vi "Configure File.vi"(8 "Error In":errorcluster, 11 "Configuration":T1={"Root Folder"=path "", "Enable Calendar Tree"=TRUE, "Maximum File Size"=15728640, "Maximum File Count"=0, "File Extension"="csv"}) -> (0 "Error Out":errorcluster)   [LabVIEW 2017, in "Toolkit.lvlib"]
doc: "All of the configurations for the default log file can be configured with this one VI instead of using VIs for each individual configuration. The individual configuration VIs are just wrappers around this VI."
uses:
  Toolkit.lvlib
  Controls/Configuration.ctl
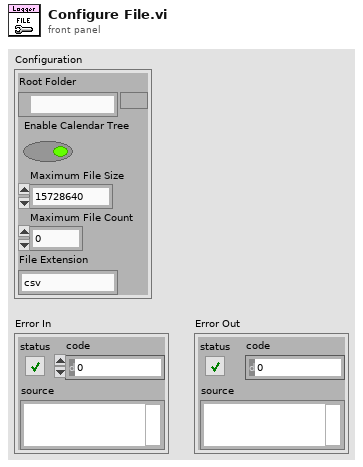
[diagram p1: front panel]
types:
  T1 = typedef "Toolkit.lvlib/Configuration.ctl" = cluster{"Root Folder":path, "Enable Calendar Tree":bool, "Maximum File Size":i64, "Maximum File Count":i32, "File Extension":string}
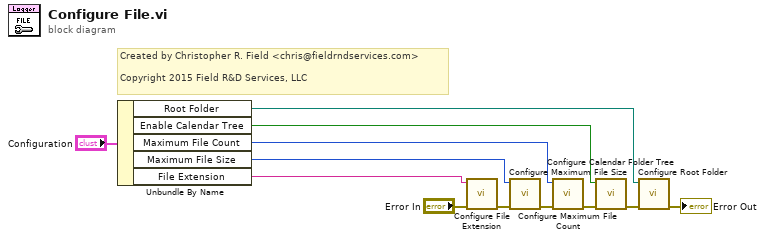
[diagram p0: block diagram]
diagram:
  # "Created by Christopher R. Field <chris@fieldrndservices.com>\n\nCopyright 2015 Field R&D Services, LLC"
  n1 = Unbundle By Name("Configuration") -> ("Root Folder"=w6:path, "Enable Calendar Tree"=w7:bool, "Maximum File Count"=w1:i32, "Maximum File Size"=w2:i64, "File Extension"=w8:string)
  n2 = call "Configure File Extension.vi"("Error In"="Error In", "File Extension"=w8) -> ("Error Out"=w3:errorcluster)  [unwired: 9 in]
  n3 = call "Configure Maximum File Size.vi"("Error In"=w3, "File Size"=w2) -> ("Error Out"=w4:errorcluster)  [unwired: 9 in]
  n4 = call "Configure Maximum File Count.vi"("Error In"=w4, "Maximum"=w1) -> ("Error Out"=w5:errorcluster)  [unwired: 9 in]
  n5 = call "Configure Calendar Folder Tree.vi"("Error In"=w5, "Enable"=w7) -> ("Error Out"=w9:errorcluster)  [unwired: 9 in]
  n6 = call "Configure Root Folder.vi"("Error In"=w9, "Root Folder"=w6) -> ("Error Out"=→"Error Out":errorcluster)  [unwired: 9 in]
